vi "SeperateChanData.vi"(0 "Input (Ch1&2)":dbl[][](array[numeric])) -> (1 "Ch1":dbl[][](array[numeric]), 2 "Ch2":dbl[][](array[numeric]))   [LabVIEW 2020]
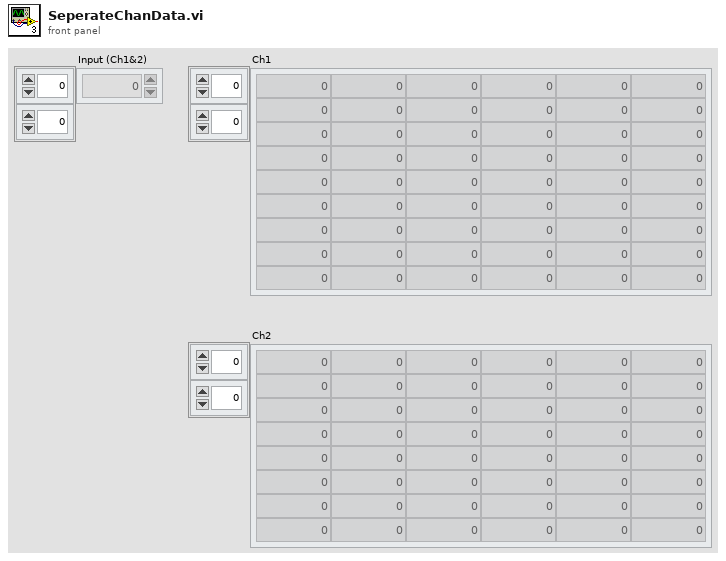
[diagram p1: front panel]
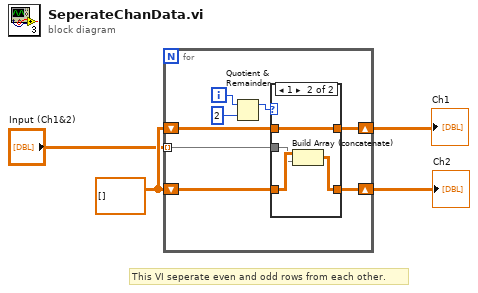
[diagram p0: block diagram]
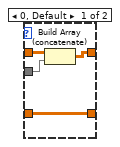
[diagram p2: hidden frame]
diagram:
  w4 = dbl[][] []
  # "This VI seperate even and odd rows from each other."
  n1 = for {
    tunnel: "Input (Ch1&2)" -> [w7] mode=indexing
    shift-right: [w6] -> w2
    shift-left: w4 -> [w9]
    shift-right: [w5] -> w3
    shift-left: w4 -> [w8]
    i -> [w12]
    n2 = Quotient & Remainder(x=w12, y=2) -> (x-y*floor(x/y)=w10:i32)  [unwired: 1 out]
    n3 = case shown="1" w10 {
      tunnel: w9 -> [w16 w20]
      tunnel: [w16 w18] -> w6
      tunnel: w8 -> [w15 w17]
      tunnel: w7 -> [w14 w19]
      tunnel: [w13 w17] -> w5
      frame 0, Default {
        n4 = Build Array (concatenate)(w15, w14) -> (w13:dbl[][])
      }
      frame 1 {
        n5 = Build Array (concatenate)(w20, w19) -> (w18:dbl[][])
      }
    }
  }
  "Ch1" <- w3
  "Ch2" <- w2
